vi "Set date and time_Core.vi"() -> ()   [LabVIEW 2011]
uses:
  <vilib>/NI_Real-Time Target Support.lvlib
panel:
  out "error out 2":errorcluster
  out "error out":errorcluster
  out "current time":timestamp
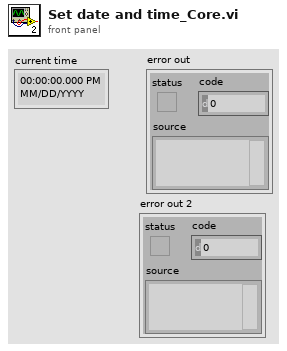
[diagram p1: front panel]
types:
  T1 = enum16{"set date", "set local time", "set UTC time"}
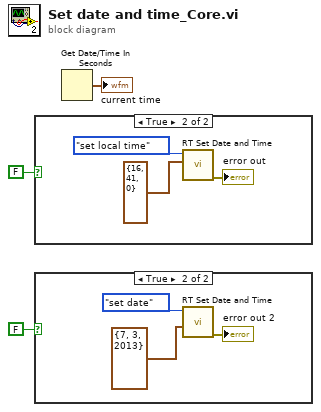
[diagram p0: block diagram]
diagram:
  n1 = case shown="True" FALSE ("ªet Time") {
    frame False {
    }
    frame True {
      n2 = call <vilib>:"RT Set Date and Time.vi"("Time"=cluster{"Hour":i32, "Minute":i32, "Second":i32} {"Hour"=16, "Minute"=41, "Second"=0}, "mode"=T1."set local time") -> ("error out"=→"error out":errorcluster)  [unwired: 9 in]
    }
  }
  n3 = case shown="True" FALSE {
    frame False {
    }
    frame True {
      n4 = call <vilib>:"RT Set Date and Time.vi"("Date"=cluster{"Month":i32, "Day":i32, "Year":i32} {"Month"=7, "Day"=3, "Year"=2013}, "mode"=T1."set date") -> ("error out"=→"error out 2":errorcluster)  [unwired: 9 in]
    }
  }
  n5 = Get Date/Time In Seconds() -> (seconds since 1Jan1904=→"current time":timestamp)
